vi "subVI_Flow Cal_Find Cal Info.vi"(1 "Flow (raw GPM)":dbl, 2 "Calibration Parsed Formulas":T1[](array[typedef])) -> (0 "Calibration Info":T1)   [LabVIEW 2018]
uses:
  Common/Controls/Parsed Formula TDEF.ctl
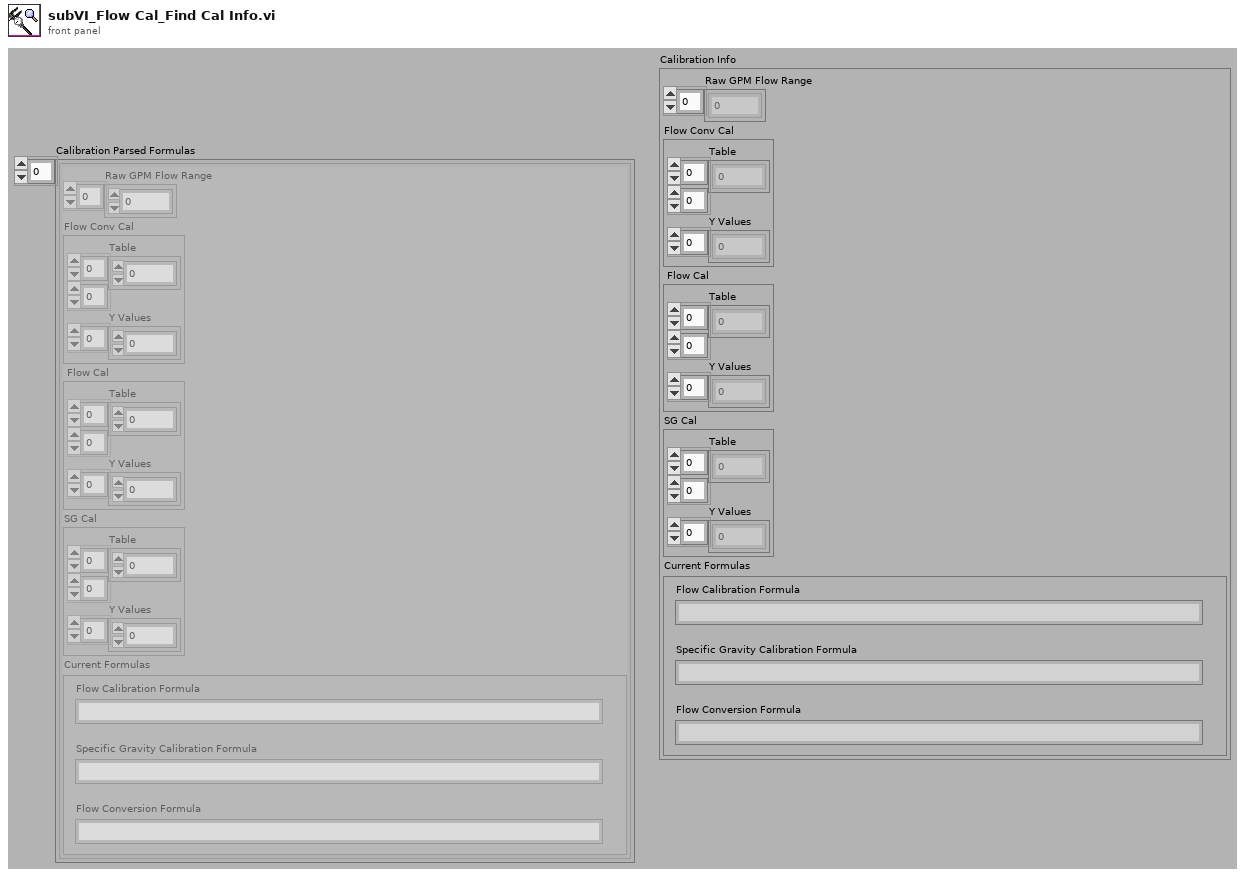
[diagram p1: front panel]
types:
  T1 = typedef "Parsed Formula TDEF.ctl" = cluster{"Raw GPM Flow Range":dbl[], "Flow Conv Cal":cluster{"Table":i32[][], "Y Values":dbl[]}, " Flow Cal":cluster{"Table":i32[][], "Y Values":dbl[]}, "SG Cal":cluster{"Table":i32[][], "Y Values":dbl[]}, "Current Formulas":cluster{"Flow Calibration Formula":string, "Specific Gravity Calibration Formula":string, "Flow Conversion Formula":string}}
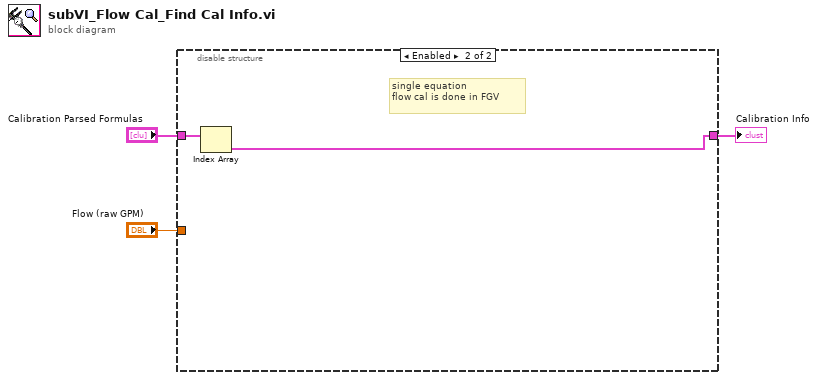
[diagram p0: block diagram]
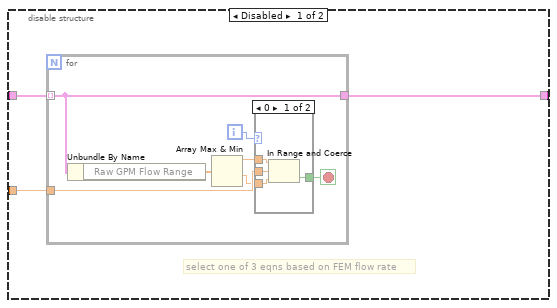
[diagram p2: hidden frame]
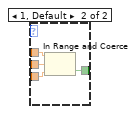
[diagram p3: hidden frame]
diagram:
  n1 = disable-structure shown="Enabled" {
    disable-tunnel: "Flow (raw GPM)" -> [w6 _]
    disable-tunnel: [w5 w22] -> w2
    disable-tunnel: "Calibration Parsed Formulas" -> [w4 w23]
    frame Disabled {
      # "select one of 3 eqns based on FEM flow rate"
      n2 = for {
        tunnel: w4 -> [w13] mode=indexing
        tunnel: [w13] -> w5
        tunnel: w6 -> [w12]
        i -> [w7]
        stop <- w8 stop-if-true
        n3 = Unbundle By Name(w13) -> ("Raw GPM Flow Range"=w9:dbl[])
        n4 = Array Max & Min(array=w9) -> (max value=w11:dbl, min value=w10:dbl)  [unwired: 2 out]
        n5 = case shown="0" w7 {
          tunnel: w12 -> [w17 w21]
          tunnel: w11 -> [w16 w20]
          tunnel: w10 -> [w15 w19]
          tunnel: [w14 w18] -> w8
          frame 0 {
            n6 = In Range and Coerce(upper limit=w16, x=w17, lower limit=w15) -> (In Range?=w14:bool)  [unwired: 1 out]
          }
          frame 1, Default {
            n7 = In Range and Coerce(upper limit=w20, x=w21, lower limit=w19) -> (In Range?=w18:bool)  [unwired: 1 out]
          }
        }
      }
    }
    frame Enabled {
      # "single equation\nflow cal is done in FGV"
      n8 = Index Array(array=w23) -> (element=w22:T1)  [unwired: 1 in]
    }
  }
  "Calibration Info" <- w2
